vi "ISPP.vi"(0 "instrument handle":refnum<k15>="PXI1Slot2 (35)", 1 "Max attempts":dbl=200.0 format="%#_13g", 2 "Step size":dbl=0.01 format="%#_13g", 5 "Lower resistance (ohm)":dbl=8586.05, 9 "Upper resistance (ohm)":dbl=9481.51, 11 "error in (no error)":errorcluster) -> (3 "SL voltage (V)":dbl=2.6, 4 "instrument handle out":refnum<k15>="PXI1Slot2 (35)", 6 "final resistance (ohm)":dbl=9301.79527642525 format="%#_6p", 8 "target hit?":bool, 10 "final current (A)":dbl=2.150122573723871e-05, 12 "BL voltage (V)":dbl=1.5, 14 "WL voltage (V)":dbl=3.12, 15 "error out":errorcluster)   [LabVIEW 2018]
panel:
  out "attempt number":i32=25
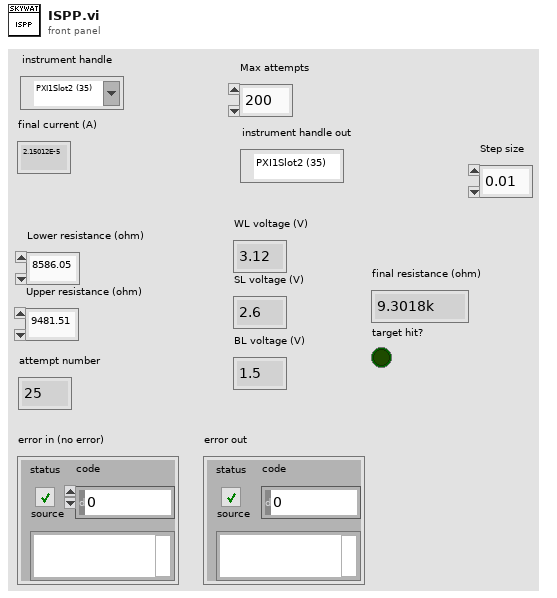
[diagram p1: front panel]
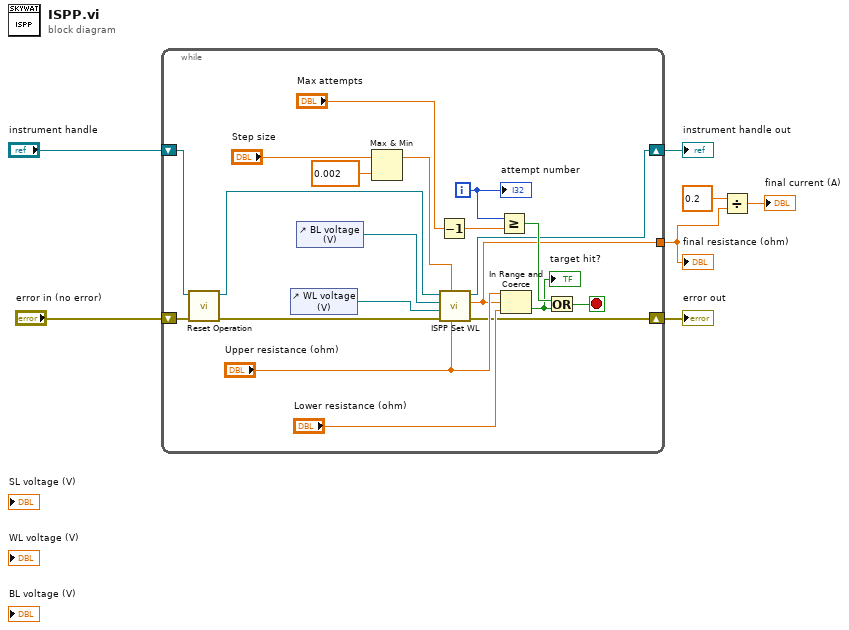
[diagram p0: block diagram]
diagram:
  n1 = while {
    shift-right: [w19] -> w6
    shift-left: "instrument handle" -> [w14]
    shift-right: [w18] -> w5
    shift-left: "error in (no error)" -> [w17]
    tunnel: [w15] -> w1
    i -> [w26]
    stop <- w27 stop-if-true
    n2 = call "Reset Operation.vi"("error in (no error)"=w17, "instrument handle"=w14) -> ("error out"=w16:errorcluster, "instrument handle out"=w13:refnum<k15>)  [unwired: 8 in]
    n3 = control-ref of="WL voltage (V)"() -> (w22:refnum<vi>)
    n4 = control-ref of="BL voltage (V)"() -> (w23:refnum<vi>)
    n5 = Max & Min(x="Step size", y=0.002) -> (max(x,y)=w8:dbl)  [unwired: 1 out]
    n6 = Decrement(x="Max attempts") -> (x-1=w11:dbl)
    n7 = call "ISPP Set WL.vi"("Target resistance (ohm)"="Upper resistance (ohm)", "Step size"=w8, "error in (no error)"=w16, "WL voltage ref"=w22, "BL voltage ref"=w23, "instrument handle"=w13) -> ("error out"=w18:errorcluster, "Final resistance (ohm)"=w15:dbl, "instrument handle out"=w19:refnum<k15>)  [unwired: 3 in]
    n8 = Greater Or Equal?(x=w26, y=w11) -> (x >= y?=w25:bool)
    n9 = In Range and Coerce(upper limit="Upper resistance (ohm)", x=w15, lower limit="Lower resistance (ohm)") -> (In Range?=w24:bool)  [unwired: 1 out]
    "target hit?" <- w24
    n10 = Or(x=w25, y=w24) -> (x .or. y?=w27:bool)
    "attempt number" <- w26
  }
  "error out" <- w5
  "instrument handle out" <- w6
  "final resistance (ohm)" <- w1
  n11 = Divide(x=0.2, y=w1) -> (x/y=→"final current (A)":dbl)
